vi "change CAD coordinates.vi"() -> ()   [LabVIEW 2019]
uses:
  <vilib>/Analysis/coordinate.llb/2D Cartesian Coordinate Rotation (Scalar).vi
  <vilib>/Analysis/NI_AALPro.lvlib
panel:
  in  "stop":bool
  in  "Rotate by angle":bool
  in  "theta (degrees)":dbl
  in  "Flip Y sign":bool
  in  "Flip X sign":bool
  in  "increase radius":bool
  in  "inc":dbl format="%#_13g"
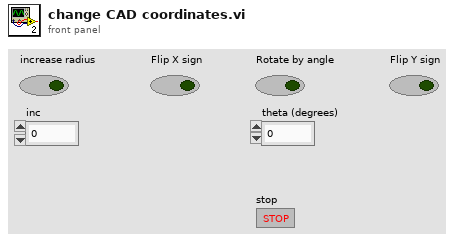
[diagram p1: front panel]
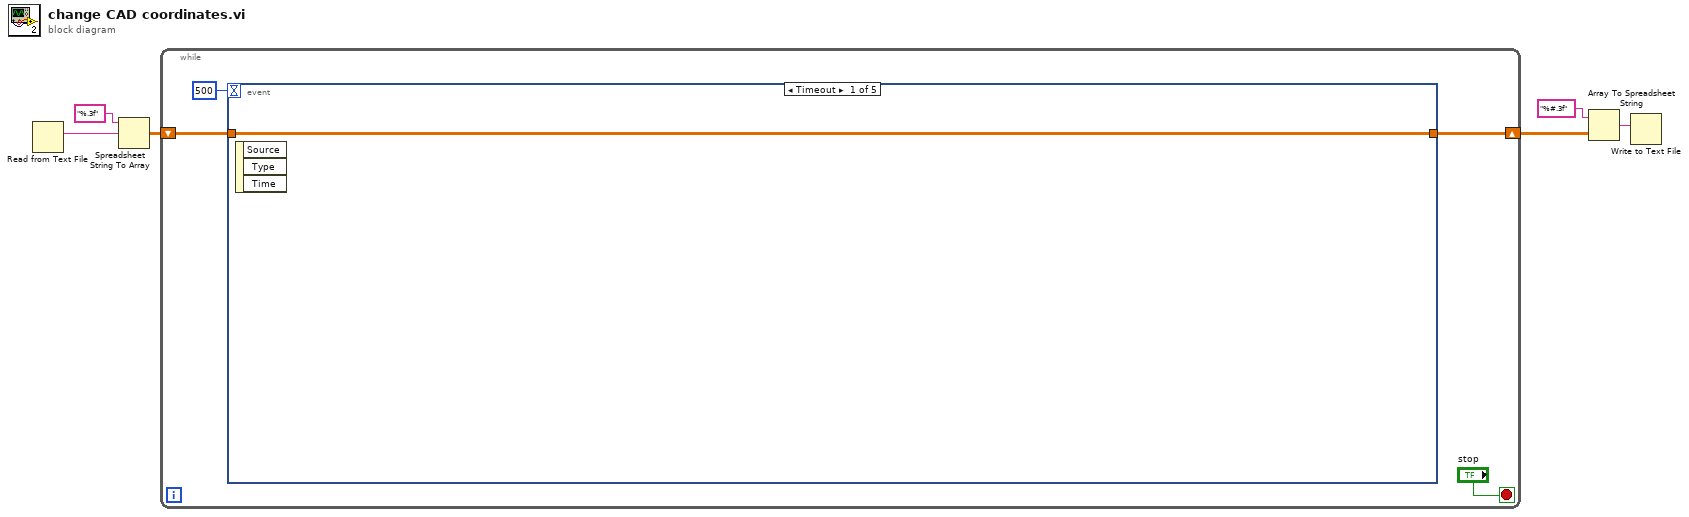
[diagram p0: block diagram]
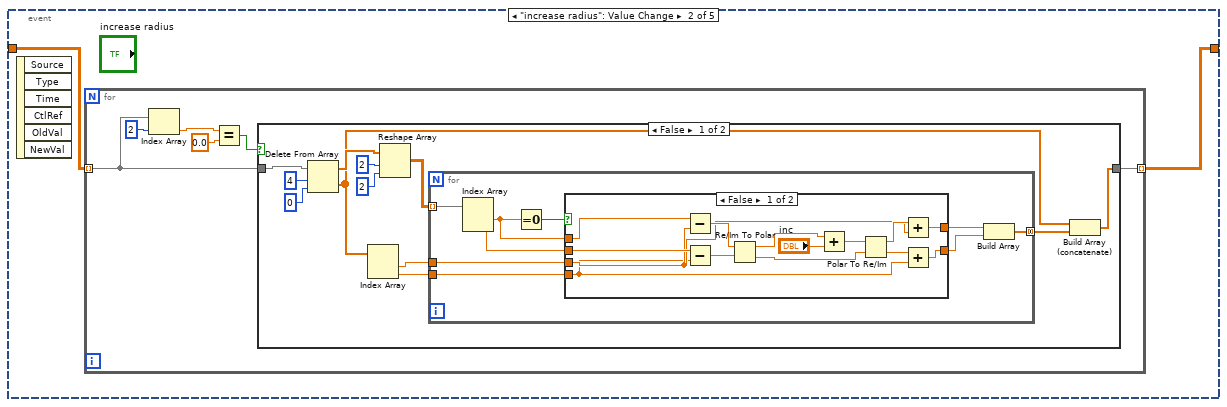
[diagram p2: hidden frame]
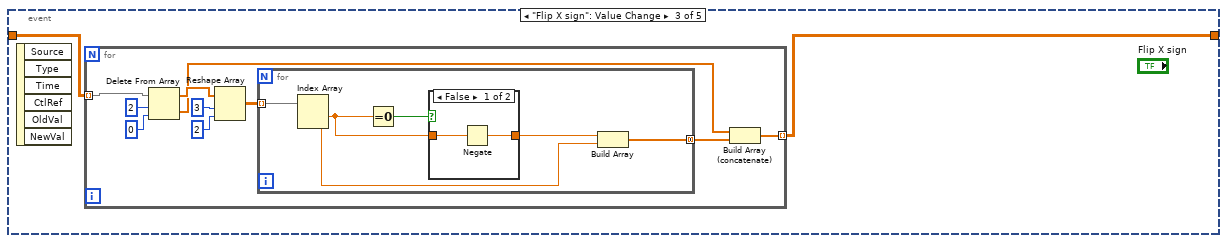
[diagram p5: hidden frame]
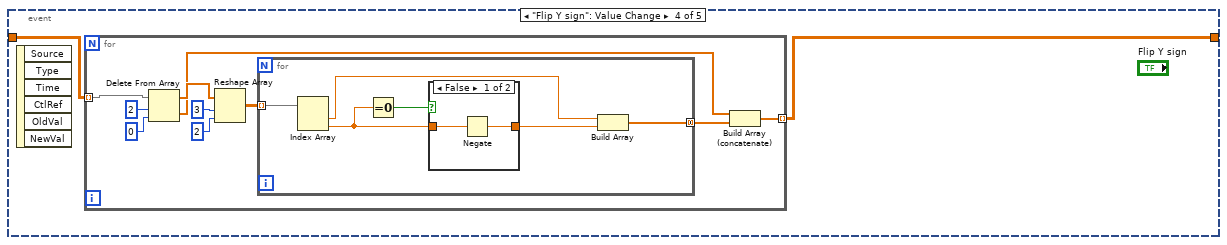
[diagram p7: hidden frame]
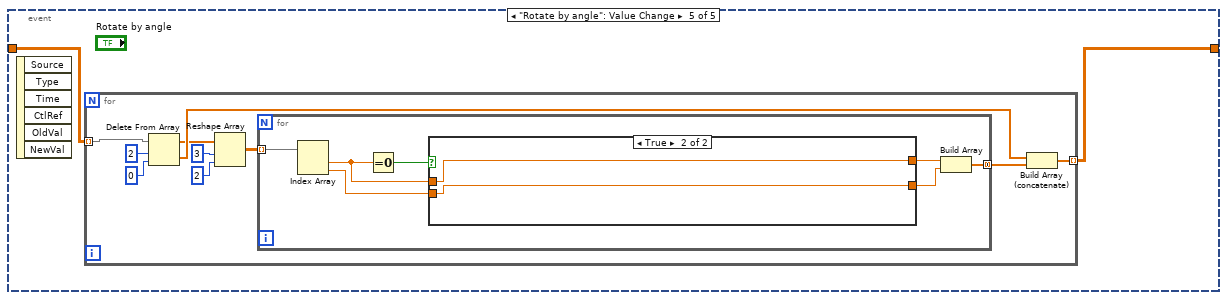
[diagram p9: hidden frame]
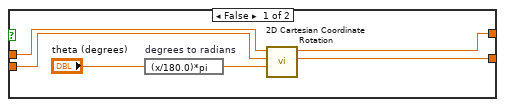
[diagram p10: hidden frame]
diagram:
  n1 = Read from Text File() -> (text=w6:string)  [unwired: 4 in, 3 out]
  n2 = Spreadsheet String To Array(format string="%.3f", spreadsheet string=w6) -> (array=w4:dbl[][])  [unwired: 2 in]
  n3 = while {
    shift-right: [w7] -> w1
    shift-left: w4 -> [w8]
    stop <- "stop" stop-if-true
    n4 = event shown="[0] Timeout" {
      selector: _ -> [_ _ _ _ _]
      dyn-events: _ -> [_ _ _ _ _]
      timeout: 500 -> [_ _ _ _ _]
      tunnel: w8 -> [w11 w13 w59 w80 w101]
      tunnel: [w11 w12 w58 w79 w100] -> w7
      event Timeout {
        n5 = event-data() -> ()  [unwired: 1 in, 3 out]
      }
      event "increase radius": Value Change {
        n6 = event-data() -> ()  [unwired: 1 in, 6 out]
        n7 = for {
          tunnel: [w17] -> w12 mode=indexing
          tunnel: w13 -> [w16] mode=indexing
          n8 = Index Array(array=w16, index=2) -> (element=w14:dbl)
          n9 = Equal?(x=w14, y=0.0) -> (x = y?=w18:bool)
          n10 = case shown="False" w18 {
            tunnel: [w20 w57] -> w17
            tunnel: w16 -> [w26 w57]
            frame False {
              n11 = Delete From Array(array=w26, length=4, index=0) -> (deleted portion=w25:dbl[], array with subset deleted=w27:dbl[])
              n12 = Index Array(array=w25) -> (element #1=w23:dbl, element #2=w22:dbl)  [unwired: 2 in]
              n13 = Reshape Array(w27, 2 ("dimension size"), 2 ("dimension size")) -> (w24:dbl[][])
              n14 = for {
                tunnel: w24 -> [w40] mode=indexing
                tunnel: w23 -> [w38]
                tunnel: w22 -> [w34]
                tunnel: [w35] -> w21 mode=concatenating
                n15 = Index Array(array=w40) -> (element #1=w32:dbl, element #2=w39:dbl)  [unwired: 2 in]
                n16 = Equal To 0?(x=w32) -> (x = 0?=w33:bool)
                n17 = case shown="False" w33 {
                  tunnel: w32 -> [w54 w56]
                  tunnel: w39 -> [w52 w55]
                  tunnel: w38 -> [w45 _]
                  tunnel: [w44 w56] -> w37
                  tunnel: w34 -> [w42 _]
                  tunnel: [w41 w55] -> w36
                  frame False {
                    n18 = Subtract(x=w54, y=w45) -> (x-y=w53:dbl)
                    n19 = Subtract(x=w52, y=w42) -> (x-y=w51:dbl)
                    n20 = Re/Im To Polar(2:w51, 3:w53) -> (0:w48:dbl, 1:w50:dbl)
                    n21 = Add(x=w50, y="inc") -> (x+y=w47:dbl)
                    n22 = Polar To Re/Im(2:w48, 3:w47) -> (0:w43:dbl, 1:w46:dbl)
                    n23 = Add(x=w46, y=w45) -> (x+y=w44:dbl)
                    n24 = Add(x=w43, y=w42) -> (x+y=w41:dbl)
                  }
                  frame True {
                  }
                }
                n25 = Build Array(w37, w36) -> (w35:dbl[])
              }
              n26 = Build Array (concatenate)(w25, w21) -> (w20:dbl[])
            }
            frame True {
            }
          }
        }
      }
      event "Flip X sign": Value Change {
        n27 = event-data() -> ()  [unwired: 1 in, 6 out]
        n28 = for {
          tunnel: w59 -> [w68] mode=indexing
          tunnel: [w69] -> w58 mode=indexing
          n29 = Delete From Array(array=w68, length=2, index=0) -> (deleted portion=w61:dbl[], array with subset deleted=w63:dbl[])
          n30 = Reshape Array(w63, 3 ("dimension size"), 2 ("dimension size")) -> (w62:dbl[][])
          n31 = for {
            tunnel: w62 -> [w75] mode=indexing
            tunnel: [w72] -> w60 mode=concatenating
            n32 = Index Array(array=w75) -> (element #1=w70:dbl, element #2=w73:dbl)  [unwired: 2 in]
            n33 = Equal To 0?(x=w70) -> (x = 0?=w71:bool)
            n34 = case shown="False" w71 {
              tunnel: w70 -> [w77 w78]
              tunnel: [w76 w78] -> w74
              frame False {
                n35 = Negate(x=w77) -> (-x=w76:dbl)
              }
              frame True {
              }
            }
            n36 = Build Array(w74, w73) -> (w72:dbl[])
          }
          n37 = Build Array (concatenate)(w61, w60) -> (w69:dbl[])
        }
      }
      event "Flip Y sign": Value Change {
        n38 = event-data() -> ()  [unwired: 1 in, 6 out]
        n39 = for {
          tunnel: w80 -> [w89] mode=indexing
          tunnel: [w90] -> w79 mode=indexing
          n40 = Delete From Array(array=w89, length=2, index=0) -> (deleted portion=w82:dbl[], array with subset deleted=w84:dbl[])
          n41 = Reshape Array(w84, 3 ("dimension size"), 2 ("dimension size")) -> (w83:dbl[][])
          n42 = for {
            tunnel: w83 -> [w96] mode=indexing
            tunnel: [w95] -> w81 mode=concatenating
            n43 = Index Array(array=w96) -> (element #1=w92:dbl, element #2=w93:dbl)  [unwired: 2 in]
            n44 = Equal To 0?(x=w93) -> (x = 0?=w94:bool)
            n45 = case shown="False" w94 {
              tunnel: [w98 w99] -> w91
              tunnel: w93 -> [w97 w99]
              frame False {
                n46 = Negate(x=w97) -> (-x=w98:dbl)
              }
              frame True {
              }
            }
            n47 = Build Array(w92, w91) -> (w95:dbl[])
          }
          n48 = Build Array (concatenate)(w82, w81) -> (w90:dbl[])
        }
      }
      event "Rotate by angle": Value Change {
        n49 = event-data() -> ()  [unwired: 1 in, 6 out]
        n50 = for {
          tunnel: w101 -> [w110] mode=indexing
          tunnel: [w111] -> w100 mode=indexing
          n51 = Delete From Array(array=w110, length=2, index=0) -> (deleted portion=w107:dbl[], array with subset deleted=w106:dbl[])
          n52 = Reshape Array(w106, 3 ("dimension size"), 2 ("dimension size")) -> (w103:dbl[][])
          n53 = for {
            tunnel: w103 -> [w115] mode=indexing
            tunnel: [w116] -> w102 mode=concatenating
            n54 = Index Array(array=w115) -> (element #1=w112:dbl, element #2=w114:dbl)  [unwired: 2 in]
            n55 = Equal To 0?(x=w112) -> (x = 0?=w113:bool)
            n56 = case shown="True" w113 {
              tunnel: [w122 w126] -> w118
              tunnel: [w121 w125] -> w117
              tunnel: w112 -> [w120 w126]
              tunnel: w114 -> [w119 w125]
              frame False {
                n57 = expression code="(x/180.0)*pi" "degrees to radians"("theta (degrees)") -> (w123:dbl)
                n58 = call-poly <vilib>:"2D Cartesian Coordinate Rotation.vi"("theta"=w123, "y"=w119, "x"=w120) -> ("y out"=w121:dbl, "x out"=w122:dbl)  [unwired: 6 in, 1 out]
              }
              frame True {
              }
            }
            n59 = Build Array(w118, w117) -> (w116:dbl[])
          }
          n60 = Build Array (concatenate)(w107, w102) -> (w111:dbl[])
        }
      }
    }
  }
  n61 = Array To Spreadsheet String(array=w1, 3:"%#.3f" ("format string")) -> (spreadsheet string=w3:string)  [unwired: 1 in]
  n62 = Write to Text File(text=w3) -> ()  [unwired: 3 in, 3 out]
